vi "pp3_trialTypes_makeWeightedCodeList.vi"(10 "Trial Replication Factor":i32=1 min=1, 11 "Trial Types":T1[](array[typedef])=[{"Trial Type Number"=1, "Trial Type"=enum."GO", "Trial Weight"=1, "Shock (mA)"=-1.0, "Duration (ms)"=250.0, "Sound Type"=enum."04 FM Sweep", "Stim P1"=2000.0, "Stim P2"=4000.0, "Stim P3"=0.0, "Stim P4"=0.0, "DAQ Amplitude (V)"=0.25}, {"Trial Type Number"=2, "Trial Type"=enum."NOGO", "Trial Weight"=1, "Shock (mA)"=-1.0, "Duration (ms)"=250.0, "Sound Type"=enum."04 FM Sweep", "Stim P1"=4000.0, "Stim P2"=2000.0, "Stim P3"=0.0, "Stim P4"=0.0, "DAQ Amplitude (V)"=0.25}] {"DAQ Amplitude (V)" min=0.0 max=5.0 format="%_4g"; "Shock (mA)" min=-1.0 max=5.0; "Trial Weight" step=1; "Duration (ms)" min=0.0 max=1.0; "Trial Type Number" min=1 max=256 step=1}) -> (3 "Weighted Code List":i32[](array[numeric]), 5 "Weighted Code List Length":i32)   [LabVIEW 2013]
uses:
  CTL_pp3g_Trial.ctl
  pp3_CTL_TrialType.ctl
  labolabo2/waveforms/WFTypes.ctl
  labolabo2/array/impl/NullArray_I.vi
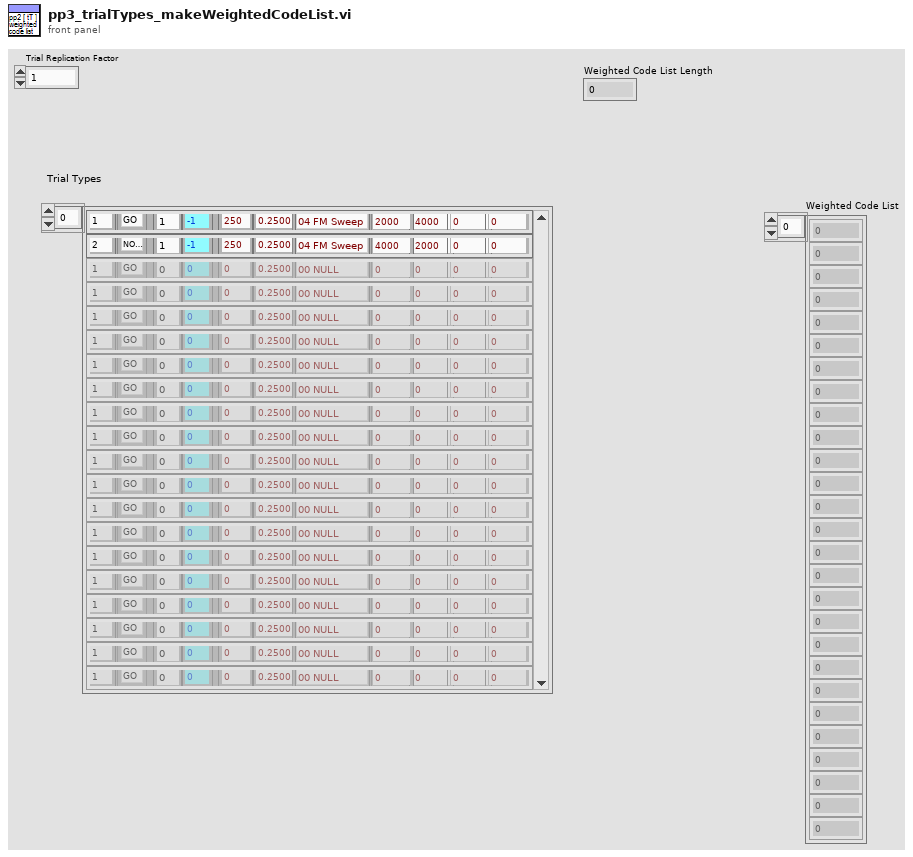
[diagram p1: front panel]
types:
  T1 = typedef "CTL_pp3g_Trial.ctl" = cluster{"Trial Type Number":i16, "Trial Type":T2, "Trial Weight":u32, "Shock (mA)":dbl, "Duration (ms)":dbl, "Sound Type":T3, "Stim P1":dbl, "Stim P2":dbl, "Stim P3":dbl, "Stim P4":dbl, "DAQ Amplitude (V)":dbl}
  T2 = typedef "pp3_CTL_TrialType.ctl" = enum16{"OFF", "GO", "NOGO", "TEST"}
  T3 = typedef "WFTypes.ctl" = enum16{"00 NULL", "01 DC", "02 Noise", "03 Pure Tone", "04 FM Sweep", "05 FM Sweep BURST"}
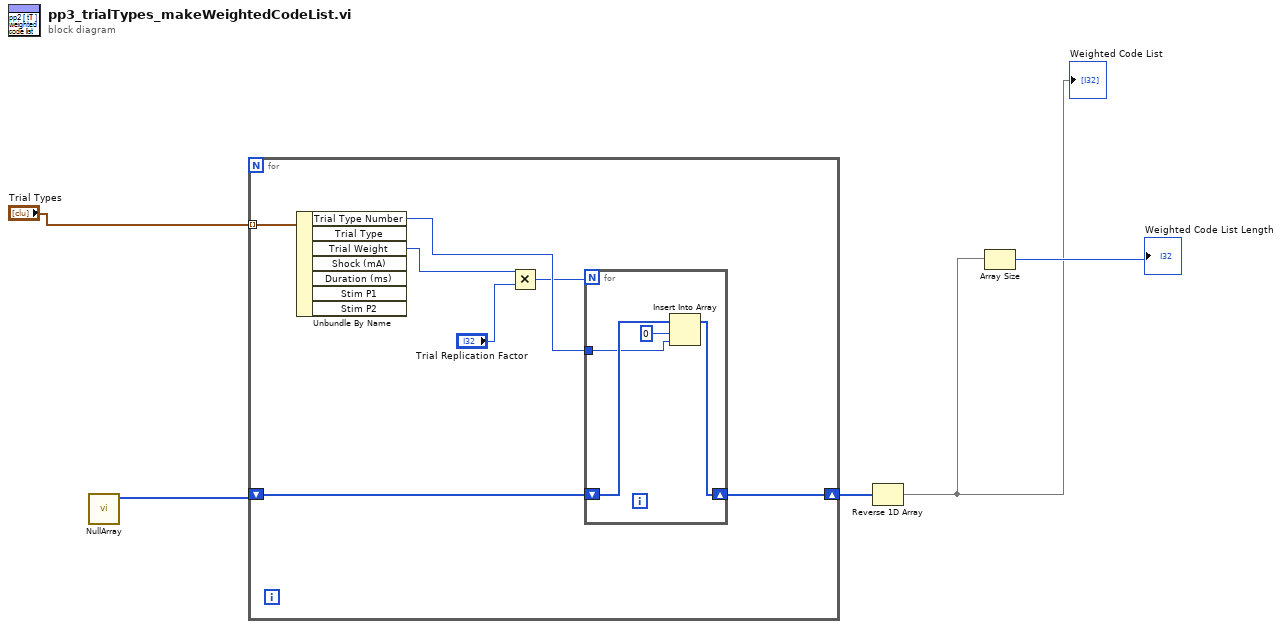
[diagram p0: block diagram]
diagram:
  n1 = call-poly "NullArray.vi"() -> ("Null Array"=w4:i32[])  [unwired: 11 in]
  n2 = for {
    tunnel: "Trial Types" -> [w10] mode=indexing
    shift-right: [w11] -> w5
    shift-left: w4 -> [w12]
    n3 = Unbundle By Name(w10) -> ("Trial Type Number"=w8:i16, "Trial Weight"=w9:u32)  [unwired: 5 out]
    n4 = Multiply(x=w9, y="Trial Replication Factor") -> (x*y=w6:u32)
    n5 = for {
      N: w6 -> [_]
      shift-right: [w13] -> w11
      shift-left: w12 -> [w15]
      tunnel: w8 -> [w14]
      n6 = Insert Into Array(array=w15, index=0, new element=w14) -> (w13:i32[])
    }
  }
  n7 = Reverse 1D Array(array=w5) -> (reversed array=w2:i32[])
  "Weighted Code List" <- w2
  n8 = Array Size(array=w2) -> (size(s)=→"Weighted Code List Length":i32)
